vi "complex_event_structure_example.vi"() -> ()   [LabVIEW 2010]
panel:
  out "Randnum":dbl
  out "x > y?":bool
  in  "Stop this VI":bool
  in  "?":bool
  # "Try to close this front panel \nwhile the VI is running."
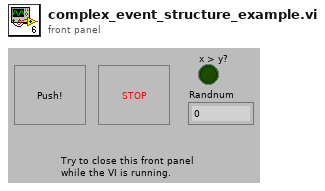
[diagram p1: front panel]
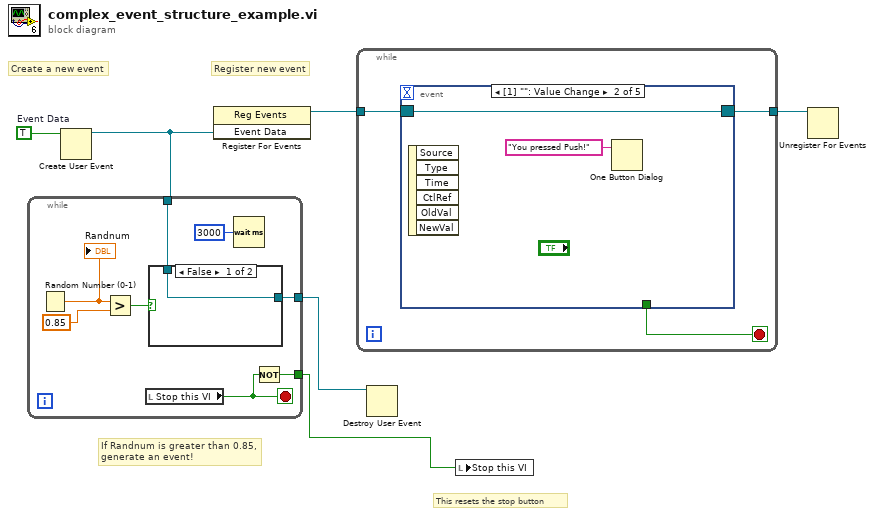
[diagram p0: block diagram]
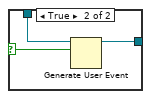
[diagram p2: hidden frame]
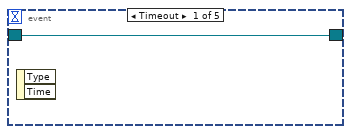
[diagram p3: hidden frame]
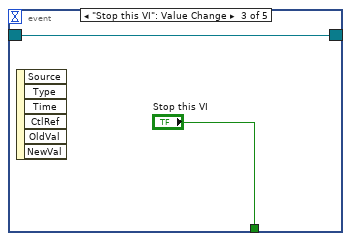
[diagram p4: hidden frame]
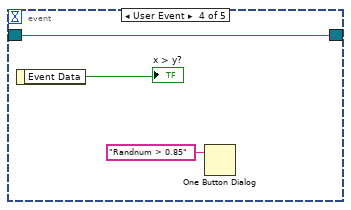
[diagram p5: hidden frame]
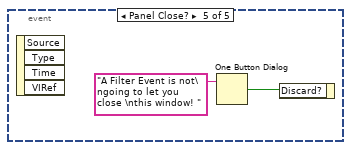
[diagram p6: hidden frame]
diagram:
  w6 = TRUE  # Event Data
  # "Register new event"
  # "Create a new event"
  # "This resets the stop button"
  # "If Randnum is greater than 0.85,\ngenerate an event!"
  n1 = Create User Event(user event datatype=w6) -> (user event=w3:refnum<user-event>)  [unwired: 1 in, 1 out]
  n2 = while {
    tunnel: w3 -> [w8]
    tunnel: [w10] -> w2
    tunnel: [w7] -> w1
    stop <- w11 stop-if-true
    n3 = Random Number (0-1)() -> (number: 0 to 1=w14:dbl)
    "Randnum" <- w14
    n4 = Greater?(x=w14, y=0.85) -> (0:w9:bool)
    n5 = local read "Stop this VI"() -> (w11:bool)
    n6 = case shown="False" w9 {
      selector: w9 -> [_ w17]
      tunnel: w8 -> [w15 w18]
      tunnel: [w15 w16] -> w7
      frame False {
      }
      frame True {
        n7 = Generate User Event(user event=w18, event data cluster=w17) -> (user event out=w16:refnum<user-event>)  [unwired: 1 in, 1 out]
      }
    }
    n8 = Wait (ms)(milliseconds to wait=u32 3000) -> ()  [unwired: 1 out]
    n9 = Not(x=w11) -> (.not. x?=w10:bool)
  }
  n10 = register-events(w3) -> (reference out=w5:refnum<event-registration>)  [unwired: 2 in, 1 out]
  n11 = while {
    tunnel: w5 -> [w20]
    tunnel: [w19] -> w4
    stop <- w21 stop-if-true
    n12 = event shown="[1] \"\": Value Change" {
      selector: w20 -> [w22 w23 w25 w29 _]
      dyn-events: [w22 w23 w25 w29 _] -> w19
      timeout: _ -> [_ _ _ _ _]
      tunnel: [_ _ "Stop this VI" _ _] -> w21
      event Timeout {
        n13 = event-data() -> ()  [unwired: 1 in, 2 out]
      }
      event Value Change {
        n14 = event-data() -> ()  [unwired: 1 in, 6 out]
        n15 = One Button Dialog(message="You pressed Push!") -> ()  [unwired: 1 in, 1 out]
      }
      event "Stop this VI": Value Change {
        n16 = event-data() -> ()  [unwired: 1 in, 6 out]
      }
      event User Event {
        n17 = event-data() -> ("Event Data"=→"x > y?":bool)  [unwired: 1 in]
        n18 = One Button Dialog(message="Randnum > 0.85") -> ()  [unwired: 1 in, 1 out]
      }
      event Panel Close? {
        n19 = event-data() -> ()  [unwired: 1 in, 4 out]
        n20 = One Button Dialog(message="A Filter Event is not\ngoing to let you close \nthis window! ") -> (true=w30:bool)  [unwired: 1 in]
        n21 = event-data("Discard?"=w30) -> ()  [unwired: 1 in, 1 out]
      }
    }
  }
  n22 = Destroy User Event(user event=w1) -> ()  [unwired: 1 in, 1 out]
  n23 = local write "Stop this VI"(w2) -> ()
  n24 = Unregister For Events(event registration refnum=w4) -> ()  [unwired: 1 in, 1 out]
